vi "Quaternion Average.vi"(8 "error in (no error)":errorcluster, 9 "Weights (Default: Empty = equal weights)":dbl[](array[numeric]), 11 "Quaternions":T1[](array[typedef])) -> (0 "error out":errorcluster, 3 "Average Quaternion":T1)   [LabVIEW 2020, in "g_ar_toolkit.ar.lvlib"]
uses:
  Quaternion.ctl
  g_ar_toolkit.ar.lvlib
  g_ar_toolkit.common/g_ar_toolkit.common.lvlib
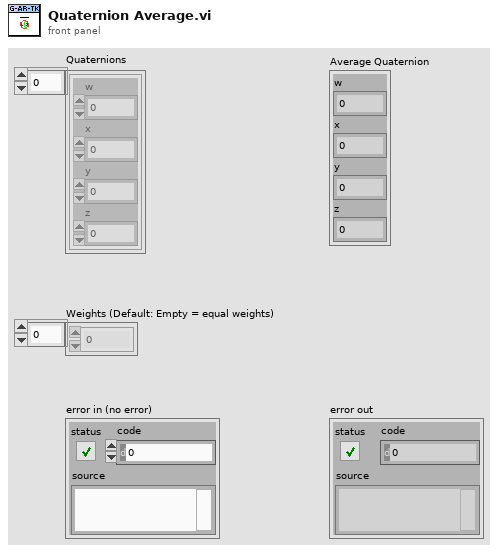
[diagram p1: front panel]
types:
  T1 = typedef "g_ar_toolkit.ar.lvlib/Quaternion.ctl" = cluster{"w":dbl, "x":dbl, "y":dbl, "z":dbl}
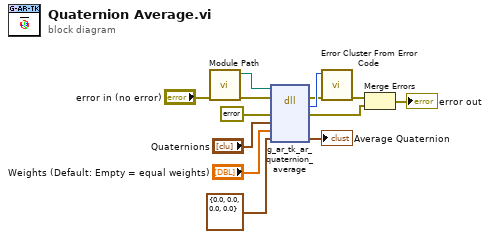
[diagram p0: block diagram]
diagram:
  n1 = call "Module Path.vi"("error in (no error)"="error in (no error)") -> ("error out"=w5:errorcluster, "Path"=w4:path)  [unwired: 9 in]
  n2 = dll-call lib="?" fn="g_ar_tk_ar_quaternion_average" ("g_ar_toolkit.*.*:g_ar_tk_image_copy")(path in=w4, error in=w5, "error_cluster"=errorcluster {"status"=FALSE, "code"=0, "source"=""} ("error constant"), "input_quaternions"="Quaternions", "Weights"="Weights (Default: Empty = equal weights)", "result_quaternion"=T1 {"w"=0.0, "x"=0.0, "y"=0.0, "z"=0.0} ("Quaternion")) -> (error out=w8:errorcluster, "MgErr"=w9:i32, "error_cluster"=w12:errorcluster, "result_quaternion"=→"Average Quaternion":T1)  [unwired: 3 in, 1 out]
  n3 = call <vilib>:"Error Cluster From Error Code.vi"("error in (no error)"=w8, "error code (0)"=w9) -> ("error out"=w10:errorcluster)  [unwired: 7 in]
  n4 = Merge Errors(w10, w12) -> (→"error out":errorcluster)
